vi "LINC Server Command Prototype.vi"() -> ()   [LabVIEW 2018, in "STEPkgDriver_LINC.lvlib"]
uses:
  STEPkgDriver_LINC.lvlib
panel:
  in  "SET_VAR_STRING":cluster{"VAL":string}={"VAL"="DEFAULT VALUE"}
  in  "SET_U8_SCALED":cluster{"VAL":u8}
  out "HANDSHAKING":cluster{"STATE":bool}
  in  "SET_ARRAY_U32":cluster{"VAL":u32[]}
  in  "ERROR":errorcluster
  in  "SET_RING":cluster{"VAL":u8} {"VAL" items=["RING_ONE"=0, "RING_TWO"=1, "RING_THREE"=2, "RING_FOUR"=4]}
  in  "SET_ENUM":T1
  in  "SET_ALL":T2 {"RING" items=["RING_ONE"=0, "RING_TWO"=1, "RING_THREE"=2, "RING_FOUR"=4]}
  in  "SET_BOOLEAN":cluster{"STATE":bool}
  in  "QUIT":cluster{"DUMMY":u8}
  in  "SET_STRING":cluster{"VAL":string}={"VAL"="DEFAULT VALUE"}
  in  "SET_NUMBER":cluster{"VAL":dbl}
  in  "COUNTER_INC":cluster{"DUMMY":u8}
  in  "COUNTER_RESET":cluster{"DUMMY":u8}
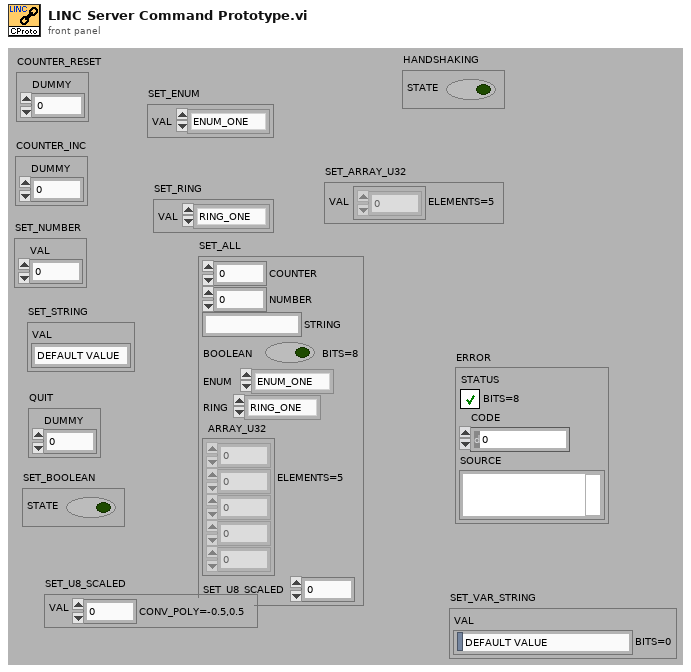
[diagram p1: front panel]
types:
  T1 = cluster{"VAL":enum8{"ENUM_ONE", "ENUM_TWO", "ENUM_THREE"}}
  T2 = cluster{"COUNTER":u32, "NUMBER":dbl, "STRING":string, "BOOLEAN":bool, "ENUM":enum8{"ENUM_ONE", "ENUM_TWO", "ENUM_THREE"}, "RING":u8, "ARRAY_U32":u32[], "SET_U8_SCALED":u8}
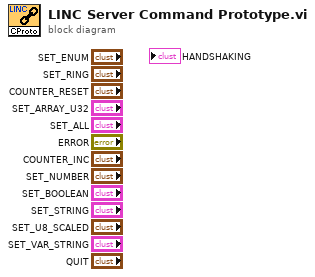
[diagram p0: block diagram]
diagram:
